vi "GlobalRight.vi"() -> ()   [LabVIEW 2020]
panel:
  in  "RightMotor":dbl
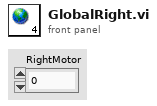
[diagram p1: front panel]
diagram:
